vi "Log Status.vi"(8 "error in (no error)":errorcluster, 11 "Message":string) -> (0 "error out":errorcluster)   [LabVIEW 2020, in "RTAF.lvlib" / "Logger Actor API.lvclass"]
uses:
  Logger Actor API.lvclass
  Base Actor/API/Actor API.lvclass/Actor API.ctl
  C:/dev/PGS/2001 - TBCM/Source/RT/RTAF/Source/RTAF/Actors/Base Actor/API/Actor API.lvclass
  Global References.vi
  Base Actor/API/Actor API.lvclass
  RTAF.lvlib
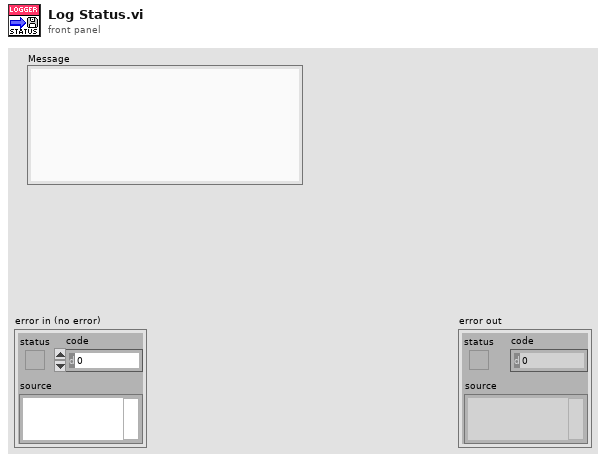
[diagram p1: front panel]
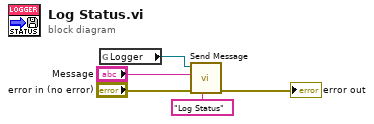
[diagram p0: block diagram]
diagram:
  n1 = global read "Global References.vi" "Logger"() -> (w1:refnum<class "Logger Actor API.lvclass">)
  n2 = call "Send Message.vi"("Name"="Log Status", "error in (no error)"="error in (no error)", "Payload"="Message", "Actor API in"=w1) -> ("error out"=→"error out":errorcluster)  [unwired: 7 in]
